vi "ANC_main.vi"() -> ()   [LabVIEW 2019]
uses:
  <vilib>/sound2/lvsound2.llb/Sound Data Format.ctl
  <vilib>/sound2/lvsound2.llb/Sampling Mode.ctl
  <vilib>/measure/madcrms.llb/Basic Averaged DC-RMS for 1 Chan.vi
  <vilib>/measure/maspectr.llb/FFT Power Spectrum and PSD for 1 Chan.vi
  <vilib>/sound2/lvsound2.llb/Sound Output Write (DBL Single).vi
  <vilib>/measure/NI_MAPro.lvlib
  Dynamic-Link Library.dll
panel:
  out "Output spectrum":cluster{"f0":dbl, "df":dbl, "magnitude":dbl[]}(graph)
  out "Error Graph":dbl[](graph)
  out "Input spectrum":cluster{"f0":dbl, "df":dbl, "magnitude":dbl[]}(graph)
  in  "UI Stop":bool
  out "SNR":dbl
  in  "mu (step size)":dbl min=0.0 max=0.1 step=0.0001
  in  "Case Choice":u16(ring) items=["Case 1: Feedforward", "Case 2: Feedback/Hybrid"]
  out "Output vs Input Graph":dbl[][](graph)
  out "Input Graph":dbl[](graph)
  out "Output Graph":dbl[](graph)
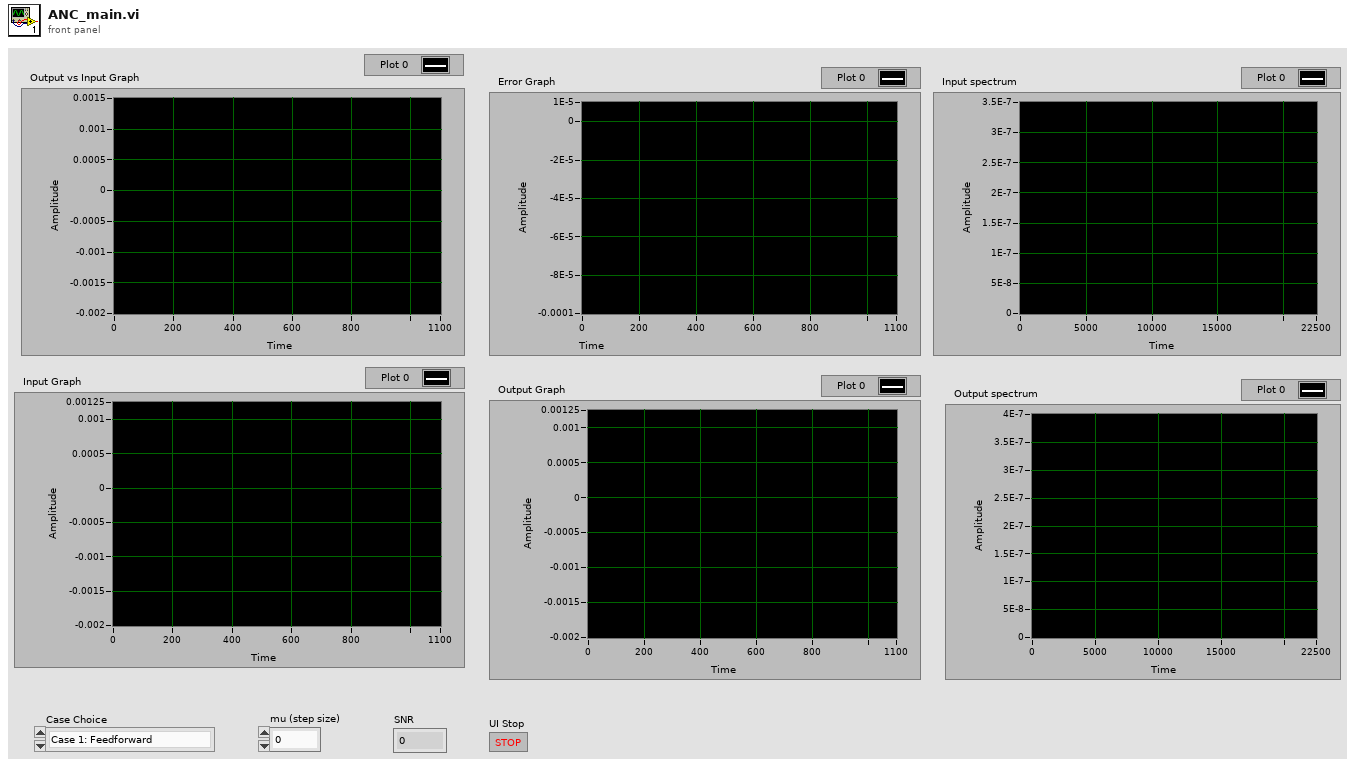
[diagram p1: front panel]
types:
  T1 = typedef "Sampling Mode.ctl" = i32
  T2 = typedef "Sound Data Format.ctl" = cluster{"sample rate (S/s)":dbl, "number of channels":i32, "bits per sample":i32}
  T3 = typedef "Sound Output Task ID.ctl" = u32
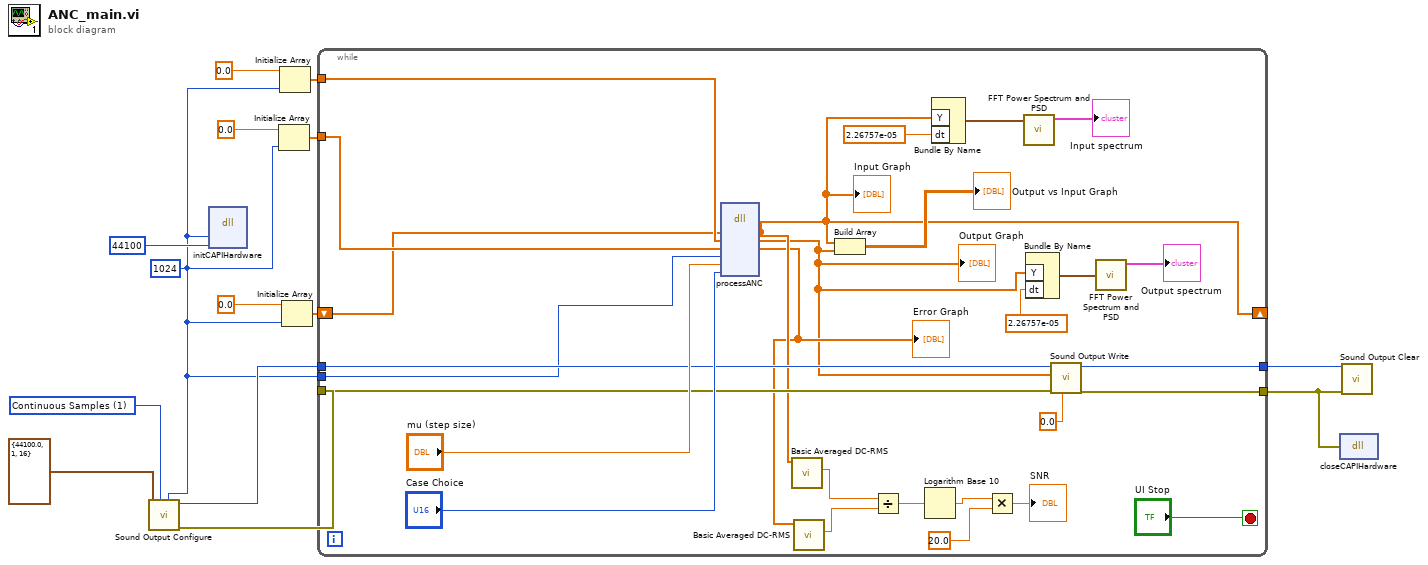
[diagram p0: block diagram]
diagram:
  w11 = T1 1 items=["Finite Samples", "Continuous Samples"] ("sample mode")
  w2 = 1024 ("number of samples/ch")
  n1 = call <vilib>:"Sound Output Configure.vi"("number of samples/ch"=w2, "sample mode"=w11, "sound format"=T2 {"sample rate (S/s)"=44100.0, "number of channels"=1, "bits per sample"=16}) -> ("error out"=w9:errorcluster, "task ID"=w10:T3)  [unwired: 7 in]
  n2 = dll-call lib="C:/Users/akdag/Desktop/EE433/433_Project/Final/EE433_ANC_Engine/EE433_ANC_Engine/Dynamic-Link Library.dll" fn="initCAPIHardware"("frameSize"=w2, "sampleRate"=44100) -> ()  [unwired: 6 in, 2 out]
  n3 = Initialize Array(0.0 ("element"), w2) -> (w6:dbl[])
  n4 = Initialize Array(0.0 ("element"), w2) -> (w13:dbl[])
  n5 = Initialize Array(0.0 ("element"), w2) -> (w1:dbl[])
  n6 = while {
    tunnel: w10 -> [w33]
    tunnel: w9 -> [w32]
    tunnel: [w31] -> w8
    tunnel: [w30] -> w4
    tunnel: w2 -> [w23]
    shift-right: [w20] -> _
    shift-left: w1 -> [w21]
    tunnel: w6 -> [w25]
    tunnel: w13 -> [w26]
    stop <- "UI Stop" stop-if-true
    n7 = dll-call lib="C:/Users/akdag/Desktop/EE433/433_Project/Final/EE433_ANC_Engine/EE433_ANC_Engine/Dynamic-Link Library.dll" fn="processANC"("mic_display"=w21, "output"=w26, "clean_error"=w25, "frameSize"=w23, "mu"="mu (step size)", "caseSelection"="Case Choice") -> ("mic_display"=w20:dbl[], "output"=w15:dbl[], "clean_error"=w19:dbl[])  [unwired: 7 in, 2 out]
    "Output Graph" <- w15
    "Input Graph" <- w20
    "Error Graph" <- w19
    n8 = call-poly <vilib>:"Basic Averaged DC-RMS.vi"("signal in"=w20) -> ("RMS value"=w40:dbl)  [unwired: 7 in, 3 out]
    n9 = call-poly <vilib>:"Basic Averaged DC-RMS.vi"("signal in"=w19) -> ("RMS value"=w39:dbl)  [unwired: 7 in, 3 out]
    n10 = Build Array(w20, w15) -> (→"Output vs Input Graph":dbl[][])
    n11 = Divide(x=w40, y=w39) -> (x/y=w38:dbl)
    n12 = Logarithm Base 10(1:w38) -> (0:w37:dbl)
    n13 = Bundle By Name("Y"=w20, "dt"=2.26757e-05) -> (w27:waveform(dbl))  [unwired: 1 in]
    n14 = Multiply(x=w37, y=20.0) -> (x*y=→"SNR":dbl)
    n15 = call-poly <vilib>:"FFT Power Spectrum and PSD.vi"("time signal"=w27) -> ("Power Spectrum / PSD"=→"Input spectrum":cluster{"f0":dbl, "df":dbl, "magnitude":dbl[]})  [unwired: 7 in, 3 out]
    n16 = Bundle By Name("Y"=w15, "dt"=2.26757e-05) -> (w16:waveform(dbl))  [unwired: 1 in]
    n17 = call-poly <vilib>:"Sound Output Write.vi"("timeout (sec)"=0.0, "error in (no error)"=w32, "data"=w15, "task ID"=w33) -> ("error out"=w30:errorcluster, "task ID out"=w31:T3)  [unwired: 6 in]
    n18 = call-poly <vilib>:"FFT Power Spectrum and PSD.vi"("time signal"=w16) -> ("Power Spectrum / PSD"=→"Output spectrum":cluster{"f0":dbl, "df":dbl, "magnitude":dbl[]})  [unwired: 7 in, 3 out]
  }
  n19 = dll-call lib="C:/Users/akdag/Desktop/EE433/433_Project/Final/EE433_ANC_Engine/EE433_ANC_Engine/Dynamic-Link Library.dll" fn="closeCAPIHardware"(error in=w4) -> ()  [unwired: 3 in, 2 out]
  n20 = call <vilib>:"Sound Output Clear.vi"("error in (no error)"=w4, "task ID"=w8) -> ()  [unwired: 9 in, 1 out]
